vi "Write to Hardware.vi"(7 "valid triggers":bool, 8 "error in":errorcluster, 9 "trigger values":dbl[](array[numeric]), 10 "Values in":dbl[](array[numeric]), 11 "Ballard ARINC-429 Tx Execution Unit in":refnum<class "Tx Scheduled Labels Execution Unit.lvclass">) -> (0 "error out":errorcluster, 1 "trigger values out":dbl[](array[numeric]), 2 "Values out":dbl[](array[numeric]), 3 "Ballard ARINC-429 Tx Execution Unit out":refnum<class "Tx Scheduled Labels Execution Unit.lvclass">)   [LabVIEW 2023, in "Ballard ARINC 429 Engine.lvlib" / "Implementation.lvlib" / "Tx Scheduled Labels Execution Unit.lvclass"]
uses:
  Tx Scheduled Labels Execution Unit.lvclass
  Tx Scheduled Labels Execution Unit.lvclass/Tx Scheduled Labels Execution Unit.ctl
  Custom Device/Write Error to System Log.vi/ca55ed61-c1f5-4d13-8aef-490b87d2cf89.vi
  Shared/Encode Parameter and Update Word (32-bit).vi/1445f95d-237d-4fc6-96b9-8992d347f513.vi
  Shared/Encode Parameter and Update Word (32-bit).vi/6b8853f0-8e5d-49e3-9391-4d3f8e5314b0.vi
  Shared/Encode Parameter and Update Word (32-bit).vi/2babc4f4-546e-4d35-846d-a4a1fbac0249.vi
  Shared/Encode Parameter and Update Word (32-bit).vi/1445f95d-237d-4fc6-96b9-8992d347f513.vi/9377bb8f-44b5-4a8f-87f1-966fd5a9edcc.vi
  Shared/Encode Parameter and Update Word (32-bit).vi/1445f95d-237d-4fc6-96b9-8992d347f513.vi/e95d9d1f-307c-44d6-9f26-c3f519a4990d.vi
  Shared/Encode Parameter and Update Word (32-bit).vi/1445f95d-237d-4fc6-96b9-8992d347f513.vi/0c23f515-4369-4514-bc3d-4444e6b437b2.vi
  Shared/Encode Parameter and Update Word (32-bit).vi/6b8853f0-8e5d-49e3-9391-4d3f8e5314b0.vi/136dcdcb-2dd3-4a4d-a796-a8f7a3f8e1ac.vi
  Shared/Encode Parameter and Update Word (32-bit).vi/6b8853f0-8e5d-49e3-9391-4d3f8e5314b0.vi/a54b505c-1216-4ef4-8378-3ceda9d188df.vi
  <vilib>/NI/NI VeriStand Encoding and Decoding/Get Bits Per Digit from Base.vi
  <vilib>/NI VeriStand/Custom Device Tools/Custom Device Utility Library/NI VeriStand - Print Debug Line.vi
  Custom Device/Custom Device.lvlib
  Hardware API/Ballard ARINC 429 Hardware API.lvlib
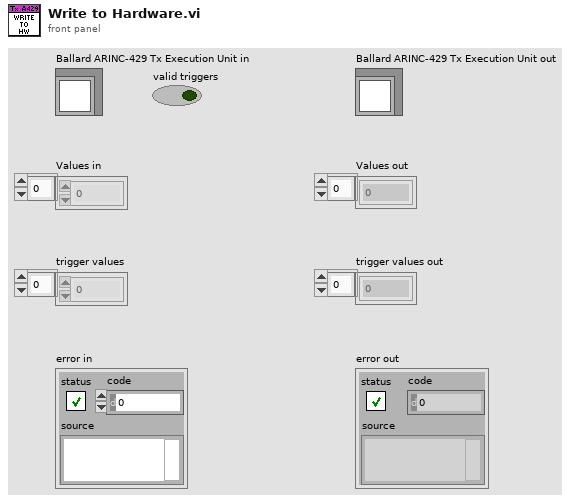
[diagram p1: front panel]
types:
  T1 = typedef "RT Hardware Channel Settings.ctl" = cluster{"channel #":u16, "channel handle":u64, "labels settings for RT":T2[]}
  T2 = typedef "RT Label Settings.ctl" = cluster{"Name":string, "xmlName":string, "label":T3, "transfer period":u32, "SDI_Enabled":bool, "SDI":u8, "parameter driver data":T4, "transfer type":T8, "has timestamp?":bool, "Label Disable/Trigger Channel Reference":T7, "Message Handle":u64, "Initialized?":bool, "Word Initial Raw Value":u32, "Label Timestamp Channel Data Reference":T9, "disabled":bool}
  T3 = typedef "Label.ctl" = u8
  T4 = typedef "RT Parameters.ctl" = cluster{"parameter definitions":T5[], "Tx parameter refs":T7[]}
  T5 = typedef "Parameter Definition.ctl" = cluster{"start index":i32, "size":i32, "encoding":T6, "signed":bool, "scale multiplier":dbl, "scale offset":dbl}
  T6 = typedef "Encoding and Decoding.lvlib/Encoding.ctl" = enum16{"BNR", "BCD", "Discrete"}
  T7 = typedef "Custom Device API.lvlib/Custom Device Item Ref.ctl" = u64
  T8 = typedef "Transfer Type.ctl" = enum16{"Scheduled", "Acyclic", "Block", "Strobe"}
  T9 = typedef "Custom Device API.lvlib/Data Reference.ctl" = i32
  T10 = typedef "Map of Values Indexes to Channel and Label Indexes.ctl" = map{i32, cluster{"channel index":i32, "label index":i32, "group values start index":i32, "values in group":i32}}
  T11 = cluster{"channel index":i32, "label index":i32, "group values start index":i32, "values in group":i32}
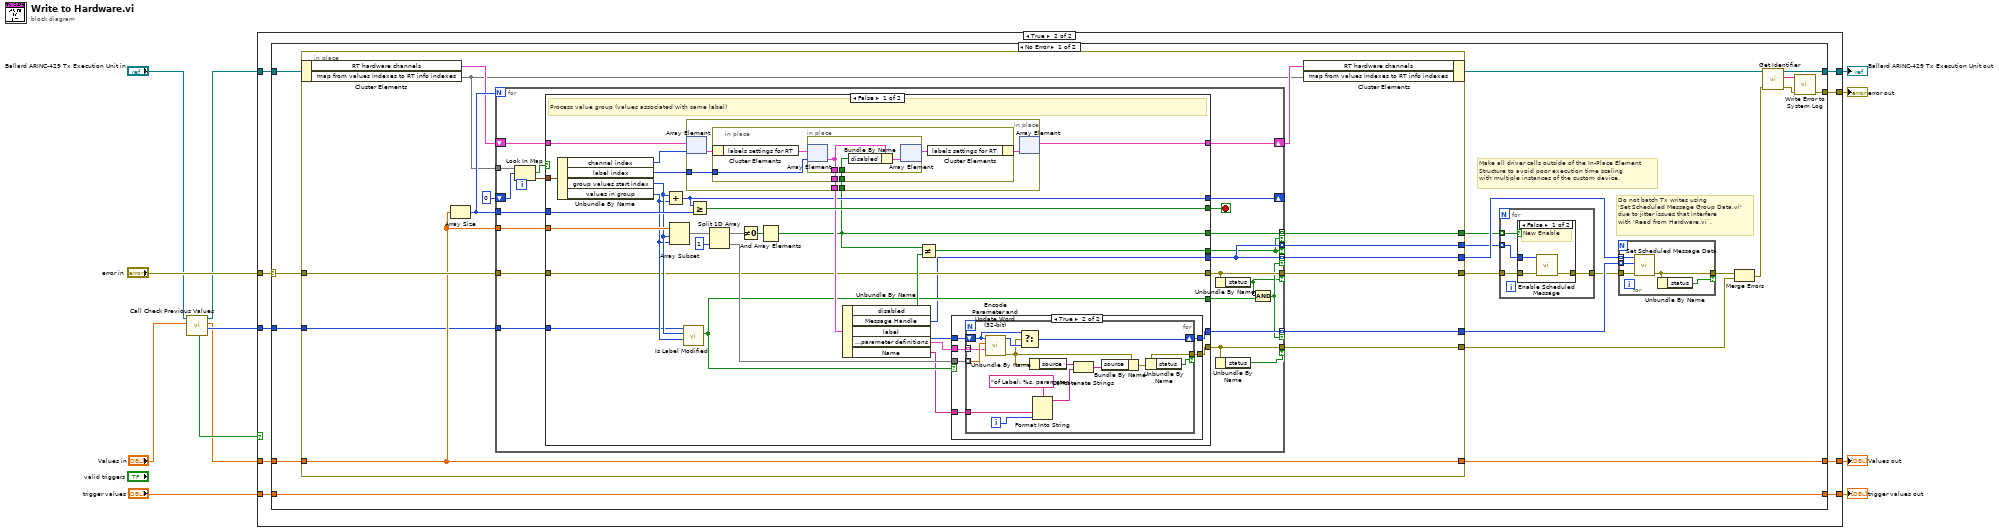
[diagram p0: block diagram]
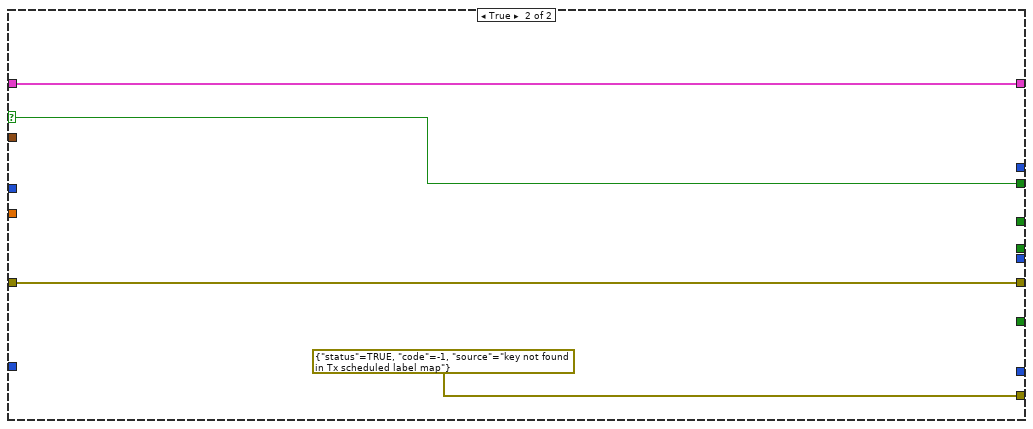
[diagram p4: hidden frame]
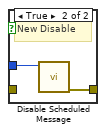
[diagram p5: hidden frame]
diagram:
  n1 = call "Call Check Previous Values.vi"("values"="Values in", "Tx Scheduled Labels Execution Unit in"="Ballard ARINC-429 Tx Execution Unit in") -> ("modified indices"=w4:i32[], "values out"=w1:dbl[], "Tx Scheduled Labels Execution Unit out"=w2:refnum<class "Tx Scheduled Labels Execution Unit.lvclass">, "values modified?"=w5:bool)  [unwired: 5 in, 1 out]
  n2 = case shown="True" w5 {
    tunnel: [w14 w25] -> w12
    tunnel: "error in" -> [w14 w24]
    tunnel: [w15 w23] -> w10
    tunnel: [w13 w22] -> w9
    tunnel: w2 -> [w13 w21]
    tunnel: [w16 w20] -> w8
    tunnel: "trigger values" -> [w16 w19]
    tunnel: w1 -> [w15 w18]
    tunnel: w4 -> [_ w17]
    frame False {
      # "If the Values in have not changed since the last call to Write to Hardware, skip the Write to Hardware step"
    }
    frame True {
      n3 = case shown="No Error" w24 {
        selector: w24 -> [w38 w165]
        tunnel: [w39 w165] -> w25
        tunnel: [w32 w164] -> w23
        tunnel: w18 -> [w45 w164]
        tunnel: [w40 w166] -> w22
        tunnel: w21 -> [w33 w166]
        tunnel: [w42 w163] -> w20
        tunnel: w19 -> [w42 w163]
        tunnel: w17 -> [w31 _]
        frame No Error {
          # "Make all driver calls outside of the In-Place Element\nStructure to avoid poor execution time scaling\nwith multiple instances of the custom device."
          # "Do not batch Tx writes using\n'Set Scheduled Message Group Data.vi'\ndue to jitter issues that interfere\nwith 'Read from Hardware.vi`."
          n4 = in-place {
            in-place-border: [w59] -> w28
            in-place-border: w45 -> [w49]
            in-place-border: [w56] -> w30
            in-place-border: [w55] -> w44
            in-place-border: [w54] -> w43
            in-place-border: w38 -> [w53]
            in-place-border: [w49] -> w32
            in-place-border: w31 -> [w48]
            in-place-border: [w47] -> w27
            in-place-border: [w46] -> w26
            n5 = in-place-cluster #1(w33) -> ("RT hardware channels"=w52:T1[], "map from values indexes to RT info indexes"=w50:T10)
            n6 = Array Size(array=w49) -> (size(s)=w57:i32)
            n7 = for {
              N: w57 -> [_]
              tunnel: w49 -> [w76]
              tunnel: [w81] -> w54 mode=indexing if=w65
              tunnel: [w62] -> w59 mode=indexing if=w65
              tunnel: w50 -> [w79]
              shift-right: [w74] -> _
              shift-left: 0 -> [w78]
              tunnel: w57 -> [w75]
              shift-right: [w71] -> w51
              shift-left: w52 -> [w80]
              tunnel: w53 -> [w70]
              tunnel: [w67] -> w56 if=w63
              tunnel: [w69] -> w55 if=w68
              tunnel: w48 -> [w66]
              tunnel: [w62] -> w46 mode=indexing if=w60
              tunnel: [w61] -> w47 mode=indexing if=w60
              stop <- w72 stop-if-true
              n8 = Look In Map(map=w79, key=w78) -> (key not found?=w73:bool, value=w77:T11)  [unwired: 1 in]
              n9 = case shown="False" w73 {
                selector: w73 -> [_ w148]
                tunnel: [w106 _] -> w81
                tunnel: w70 -> [w87 w146]
                tunnel: [w91 errorcluster {"status"=TRUE, "code"=-1, "source"="key not found in Tx scheduled label map"} ("error in")] -> w69
                tunnel: [w86 _] -> w62
                tunnel: w80 -> [w95 w147]
                tunnel: w77 -> [w110 _]
                tunnel: w76 -> [w109 _]
                tunnel: w75 -> [w108 _]
                tunnel: [w96 _] -> w74
                tunnel: [w107 w148] -> w72
                tunnel: [w93 w147] -> w71
                tunnel: [w87 w146] -> w67
                tunnel: w66 -> [w83 _]
                tunnel: [w88 _] -> w64
                tunnel: [w85 _] -> w60
                tunnel: [w84 _] -> w61
                frame False {
                  # "Process value group (values associated with same label)"
                  n10 = Unbundle By Name(w110) -> ("channel index"=w94:i32, "label index"=w97:i32, "group values start index"=w90:i32, "values in group"=w89:i32)
                  n11 = Add(x=w90, y=w89) -> (x+y=w96:i32)
                  n12 = Array Subset(array=w109, index=w90, length=w89) -> (w104:dbl[])
                  n13 = call "Is Label Modified.vi"("number of parameters"=w89, "initial index"=w90, "modified indices"=w83) -> ("label modified"=w88:bool)  [unwired: 8 in]
                  n14 = Greater Or Equal?(x=w96, y=w108) -> (x >= y?=w107:bool)
                  n15 = Split 1D Array(array=w104, index=1) -> (first subarray=w103:dbl[], second subarray=w92:dbl[])
                  n16 = Not Equal To 0?(x=w103) -> (x != 0?=w102:bool[])
                  n17 = And Array Elements(Boolean array=w102) -> (logical AND=w84:bool)
                  n18 = in-place {
                    in-place-border: [w136] -> w98
                    in-place-border: w84 -> [w135]
                    in-place-border: w97 -> [w134]
                    n19 = in-place-array #2(w95, w94) -> (w132:T1)
                    n20 = in-place {
                      in-place-border: [w141] -> w136
                      in-place-border: w135 -> [w140]
                      in-place-border: w134 -> [w139]
                      n21 = in-place-cluster #3(w132) -> ("labels settings for RT"=w138:T2[])
                      n22 = in-place {
                        in-place-border: [w143] -> w141
                        in-place-border: w140 -> [w144]
                        n23 = in-place-array #4(w138, w139) -> (w143:T2)
                        n24 = Bundle By Name(cluster=w143, "disabled"=w144) -> (w142:T2)
                        n25 = in-place-array #4(w142) -> (w137:T2[])  [unwired: 1 out]
                      }
                      n26 = in-place-cluster #3("labels settings for RT"=w137) -> (w133:T1)
                    }
                    n27 = in-place-array #2(w133) -> (w93:T1[])  [unwired: 1 out]
                  }
                  n28 = Unbundle By Name(w98) -> ("disabled"=w99:bool, "Message Handle"=w86:u64, "label"=w100:T3, "parameter driver data.parameter definitions"=w101:T5[], "Name"=w82:string)
                  n29 = Not Equal?(x=w84, y=w99) -> (x != y?=w85:bool)
                  n30 = case shown="True" w88 {
                    tunnel: [w111 w117] -> w106
                    tunnel: w101 -> [_ w116]
                    tunnel: w100 -> [w111 w115]
                    tunnel: w92 -> [_ w114]
                    tunnel: [_ w113] -> w91
                    tunnel: w82 -> [_ w112]
                    frame False {
                    }
                    frame True {
                      n31 = for {
                        tunnel: w114 -> [w131] mode=indexing
                        shift-right: [w128] -> w117
                        shift-left: w115 -> [w129]
                        tunnel: w116 -> [w130] mode=indexing
                        tunnel: [w121] -> w113 if=w126
                        tunnel: w112 -> [w118]
                        i -> [w119]
                        n32 = call "Encode Parameter and Update Word (32-bit).vi"("parameter definition"=w130, "parameter value"=w131, "word in"=w129) -> ("error out"=w120:errorcluster, "word out"=w127:u32)  [unwired: 7 in]
                        n33 = Select(t=w129, s=w120, f=w127) -> (s? t:f=w128:u32)
                        n34 = Unbundle By Name(w120) -> ("source"=w125:string)
                        n35 = Format Into String(format string="of Label: %s, parameter #%d", w118, w119) -> (resulting string=w122:string)  [unwired: 2 in, 1 out]
                        n36 = Concatenate Strings(w125, w122) -> (w124:string)
                        n37 = Bundle By Name(cluster=w120, "source"=w124) -> (w121:errorcluster)
                        n38 = Unbundle By Name(w121) -> ("status"=w126:bool)
                      }
                    }
                  }
                }
                frame True {
                }
              }
              n39 = Unbundle By Name(w67) -> ("status"=w63:bool)
              n40 = Unbundle By Name(w69) -> ("status"=w68:bool)
              n41 = Compound Arithmetic op=AND(invert w63, w64) -> (w65:bool)
            }
            n42 = in-place-cluster #1("RT hardware channels"=w51, "map from values indexes to RT info indexes"=w50) -> (w36:refnum<class "Tx Scheduled Labels Execution Unit.lvclass">)
          }
          n43 = for {
            tunnel: w30 -> [w152]
            tunnel: [w151] -> w29
            tunnel: w27 -> [w150] mode=indexing
            tunnel: w26 -> [w149] mode=indexing
            n44 = case shown="False" w150 {
              tunnel: w149 -> [w155 w157]
              tunnel: [w154 w156] -> w151
              tunnel: w152 -> [w153 _]
              frame False {
                # "New Enable"
                n45 = call "Enable Scheduled Message.vi"("error in (no error)"=w153, "message handle in"=w155) -> ("error out"=w154:errorcluster)  [unwired: 8 in, 1 out]
              }
              frame True {
                # "New Disable"
                n46 = call "Disable Scheduled Message.vi"("message handle in"=w157) -> ("error out"=w156:errorcluster)  [unwired: 9 in, 1 out]
              }
            }
          }
          n47 = for {
            tunnel: w28 -> [w160] mode=indexing
            tunnel: w43 -> [w162] mode=indexing
            tunnel: w29 -> [w161]
            tunnel: [w159] -> w37 if=w158
            n48 = call "Set Scheduled Message Data.vi"("error in (no error)"=w161, "value"=w162, "message handle in"=w160) -> ("error out"=w159:errorcluster)  [unwired: 7 in, 1 out]
            n49 = Unbundle By Name(w159) -> ("status"=w158:bool)
          }
          n50 = Merge Errors(w37, w44) -> (w35:errorcluster)
          n51 = call-dynamic "Get Identifier.vi"("error in"=w35, "Ballard ARINC-429 Execution Unit in"=w36) -> ("error out"=w34:errorcluster, "identifier"=w41:string, "Ballard ARINC-429 Execution Unit out"=w40:refnum<class "Tx Scheduled Labels Execution Unit.lvclass">)  [unwired: 7 in]
          n52 = call "Write Error to System Log.vi"("error in"=w34, "identifier"=w41) -> ("error out"=w39:errorcluster)  [unwired: 9 in]
        }
        frame Error {
        }
      }
    }
  }
  "error out" <- w12
  "Ballard ARINC-429 Tx Execution Unit out" <- w9
  "Values out" <- w10
  "trigger values out" <- w8
